vi "GitDiffFiles.vi"(8 "error in (no error)":errorcluster, 9 "New File":path=path "", 10 "Old File":path=path "", 11 "Git exec":string="git") -> (0 "error out":errorcluster, 1 "New File out":path, 2 "Response":string, 3 "Git exec out":string="git", 4 "Differ":bool)   [LabVIEW 2013]
uses:
  GitCmd.vi
  <vilib>/Utility/error.llb/General Error Handler.vi
  GitUtils/PathtoDirPath.vi
  <vilib>/Platform/system.llb/System Exec.vi
  <vilib>/Utility/error.llb/Error Cluster From Error Code.vi
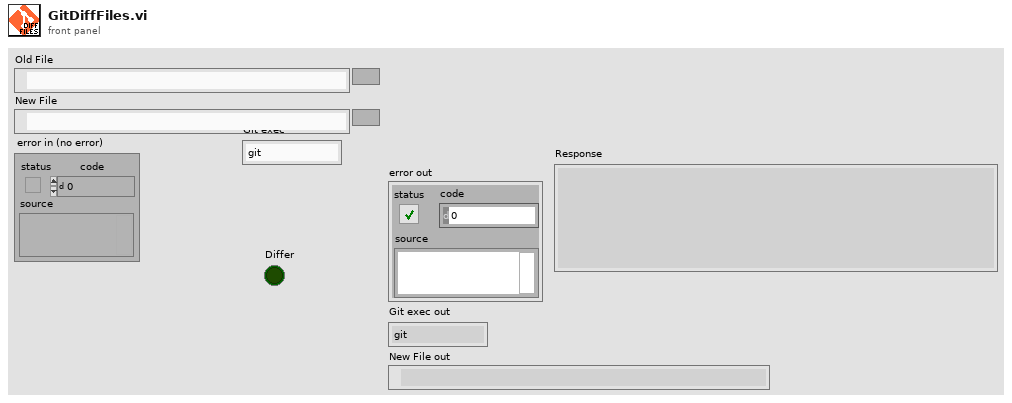
[diagram p1: front panel]
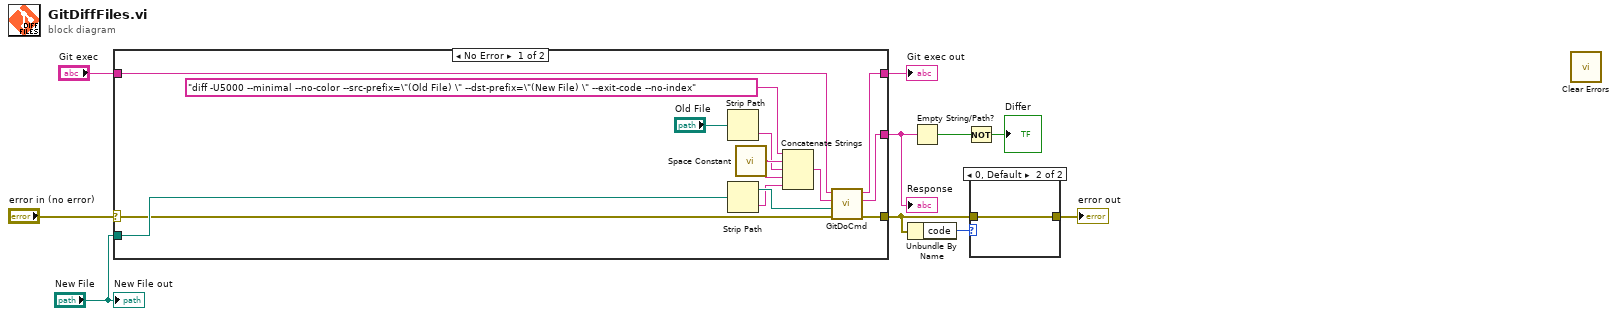
[diagram p0: block diagram]
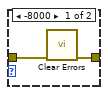
[diagram p2: hidden frame]
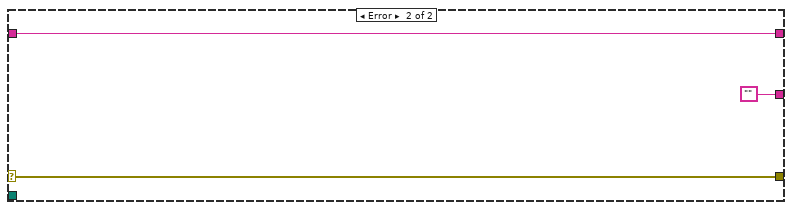
[diagram p3: hidden frame]
diagram:
  n1 = case shown="No Error" "error in (no error)" {
    selector: "error in (no error)" -> [w18 w25]
    tunnel: "Git exec" -> [w22 w24]
    tunnel: "New File" -> [w23 _]
    tunnel: [w20 ""] -> w6
    tunnel: [w17 w25] -> w2
    tunnel: [w21 w24] -> w7
    frame No Error {
      n2 = Strip Path(path="Old File") -> (name=w11:string)  [unwired: 1 out]
      n3 = Strip Path(path=w23) -> (stripped path=w19:path, name=w14:string)
      n4 = call <vilib>:"Space Constant.vi"() -> ("String"=w16:string)
      n5 = Concatenate Strings("diff -U5000 --minimal --no-color --src-prefix=\"(Old File) \" --dst-prefix=\"(New File) \" --exit-code --no-index" ("string"), w16, w11, w16, w14) -> (w13:string)
      n6 = call "GitDoCmd.vi"("error in (no error)"=w18, "Working Path"=w19, "Git command"=w13, "Git exec"=w22) -> ("error out"=w17:errorcluster, "Returned stdout"=w20:string, "Git exec out"=w21:string)  [unwired: 3 in, 1 out]
    }
    frame Error {
    }
  }
  "Response" <- w6
  "Git exec out" <- w7
  n7 = Unbundle By Name(w2) -> ("code"=w1:i32)
  n8 = Empty String/Path?(string/path=w6) -> (empty?=w5:bool)
  n9 = Not(x=w5) -> (.not. x?=→"Differ":bool)
  n10 = case shown="0, Default" w1 {
    tunnel: [w27 w29] -> w3
    tunnel: w2 -> [w28 w29]
    frame -8000 {
      n11 = call <vilib>:"Clear Errors.vi"("error in (no error)"=w28) -> ("error out"=w27:errorcluster)  [unwired: 6 in]
    }
    frame 0, Default {
    }
  }
  "error out" <- w3
  n12 = call <vilib>:"Clear Errors.vi"() -> ()  [unwired: 7 in, 1 out]
  "New File out" <- "New File"
